vi "PGPASS.default path.vi"(8 "error in (no error)":errorcluster) -> (0 "error out":errorcluster, 3 "PGPASS path":path)   [LabVIEW 2019, in "PGPASS.lvlib"]
doc: "Returns the path to the .pgpass file in a user's home directory.\n\nOn Microsoft Windows the file is named %APPDATA%\\postgresql\\pgpass.conf (where %APPDATA% refers to the Application Data subdirectory in the user's profile).\n\nMore information: https://www.postgresql.org/docs/current/libpq-pgpass.html"
uses:
  PGPASS.lvlib
  <vilib>/Utility/sysdir.llb/System Directory Type.ctl
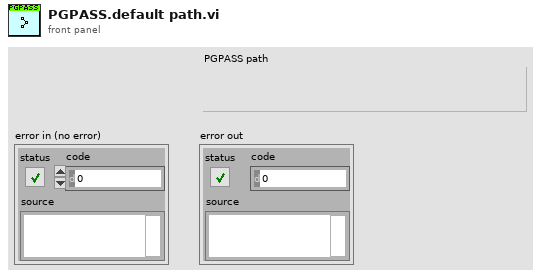
[diagram p1: front panel]
types:
  T1 = typedef "System Directory Type.ctl" = i32
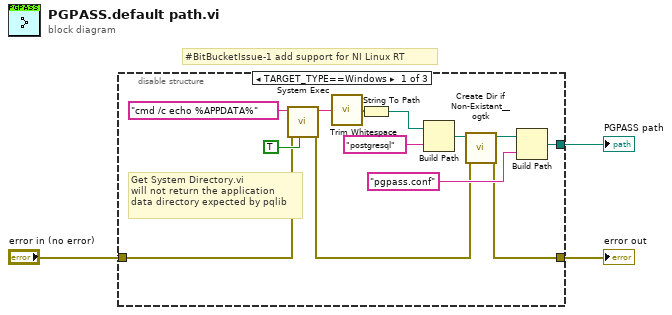
[diagram p0: block diagram]
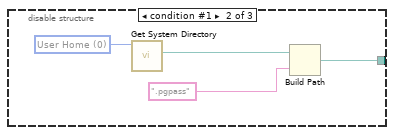
[diagram p2: hidden frame]
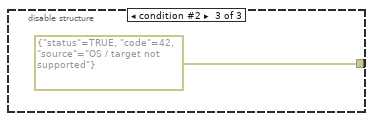
[diagram p3: hidden frame]
diagram:
  # "#BitBucketIssue-1 add support for NI Linux RT"
  n1 = disable-structure shown="TARGET_TYPE==Windows" {
    disable-tunnel: [w14 w17 _] -> w1
    disable-tunnel: [w11 _ errorcluster {"status"=TRUE, "code"=42, "source"="OS / target not supported"} ("error in (no error)")] -> w2
    disable-tunnel: "error in (no error)" -> [w4 _ _]
    frame condition #0 (active) {
      # "Get System Directory.vi\nwill not return the application\ndata directory expected by pqlib"
      n2 = call <vilib>:"System Exec.vi"("run minimized? (F)"=TRUE, "error in (no error)"=w4, "command line"="cmd /c echo %APPDATA%") -> ("error out"=w5:errorcluster, "standard output"=w7:string)  [unwired: 5 in, 2 out]
      n3 = call <vilib>:"Trim Whitespace.vi"("string"=w7) -> ("trimmed string"=w6:string)  [unwired: 1 in]
      n4 = String To Path(string=w6) -> (path=w9:path)
      n5 = Build Path(base path=w9, name or relative path="postgresql") -> (appended path=w13:path)
      n6 = call <userlib>:"Create Dir if Non-Existant__ogtk.vi"("error in (no error)"=w5, "Directory Path"=w13) -> ("error out"=w11:errorcluster, "dup Directory Path"=w12:path)  [unwired: 7 in, 1 out]
      n7 = Build Path(base path=w12, name or relative path="pgpass.conf") -> (appended path=w14:path)
    }
    frame condition #1 {
      w20 = T1 0 items=["User Home"=0, "User Desktop"=1, "User Documents"=2, "User Application Data"=3, "User Preferences"=4, "User Temporary"=5, "Public Documents"=6, "Public Application Data"=7, "Public Preferences"=8, "Public Cache"=13, "System Core Libraries"=9, "System Installed Libraries"=10, "Application Files"=11, "Boot Volume Root"=12] ("system directory type")
      n8 = call <vilib>:"Get System Directory.vi"("system directory type"=w20) -> ("system directory"=w18:path)  [unwired: 10 in]
      n9 = Build Path(base path=w18, name or relative path=".pgpass") -> (appended path=w17:path)
    }
    frame condition #2 {
    }
  }
  "error out" <- w2
  "PGPASS path" <- w1
